vi "Sweep_Test_pass_fail.vi"() -> ()   [LabVIEW 2026]
panel:
  out "Fail Count":dbl
  out "Overall PASS":bool
  in  "Gain Max (dB)":dbl
  in  "Gain Min (dB)":dbl
  out "Gain vs Frequency":cluster{dbl[], dbl[]}(graph)
  in  "Step (MHz)":dbl
  in  "Stop (MHz)":dbl
  in  "Start (MHz)":dbl
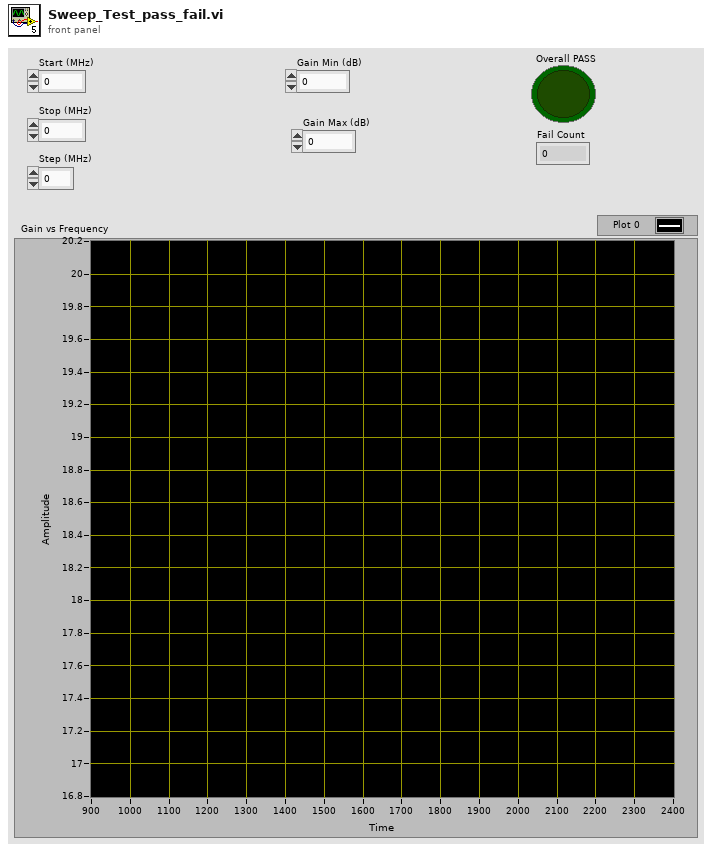
[diagram p1: front panel]
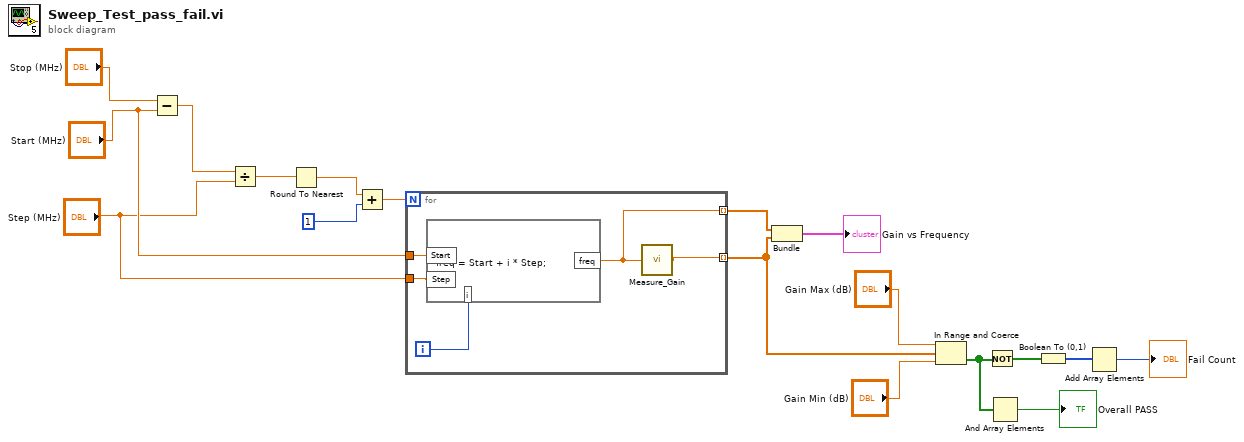
[diagram p0: block diagram]
diagram:
  n1 = Subtract(x="Stop (MHz)", y="Start (MHz)") -> (x-y=w17:dbl)
  n2 = Divide(x=w17, y="Step (MHz)") -> (x/y=w16:dbl)
  n3 = Round To Nearest(number=w16) -> (nearest integer value=w15:dbl)
  n4 = Add(x=w15, y=1) -> (x+y=w13:dbl)
  n5 = for {
    N: w13 -> [_]
    tunnel: "Start (MHz)" -> [w23]
    tunnel: "Step (MHz)" -> [w22]
    tunnel: [w20] -> w8 mode=indexing
    tunnel: [w19] -> w10 mode=indexing
    i -> [w21]
    n6 = formula code="freq = Start + i * Step;"("Start"=w23, "Step"=w22, "i"=w21) -> ("freq"=w19:dbl)
    n7 = call "Measure_Gain.vi"("Frequency (MHz)"=w19) -> ("Gain (dB)"=w20:dbl)
  }
  n8 = Bundle(w10, w8) -> (→"Gain vs Frequency":cluster{dbl[], dbl[]})  [unwired: 1 in]
  n9 = In Range and Coerce(upper limit="Gain Max (dB)", x=w8, lower limit="Gain Min (dB)") -> (In Range?=w2:bool[])  [unwired: 1 out]
  n10 = Not(x=w2) -> (.not. x?=w5:bool[])
  n11 = And Array Elements(Boolean array=w2) -> (logical AND=→"Overall PASS":bool)
  n12 = Boolean To (0,1)(Boolean=w5) -> (0, 1=w4:i16[])
  n13 = Add Array Elements(numeric array=w4) -> (sum=→"Fail Count":i16)
